vi "Set Configuration.vi"(8 "error in (no error)":errorcluster, 11 "Output Signal in":refnum<class "Output Signal.lvclass">) -> (0 "error out":errorcluster, 3 "Output Signal out":refnum<class "Output Signal.lvclass">)   [LabVIEW 2015, in "Output Signal.lvclass"]
uses:
  Output Signal.lvclass
  IO Class/Direction.ctl
  IO Class/IO Class.lvclass
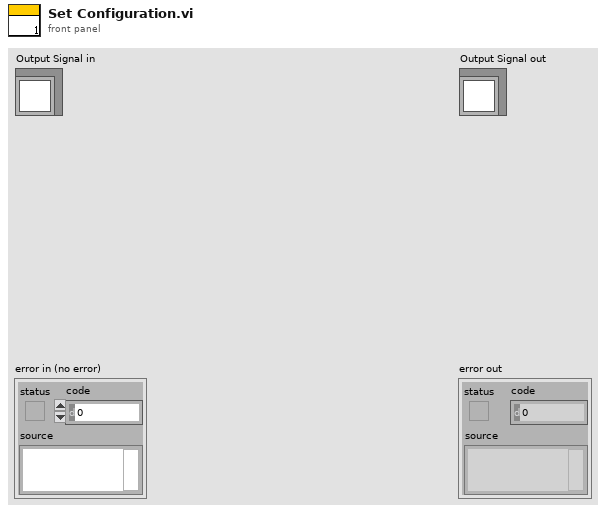
[diagram p1: front panel]
types:
  T1 = typedef "IO Class.lvclass/Direction.ctl" = cluster{"Direction":string}
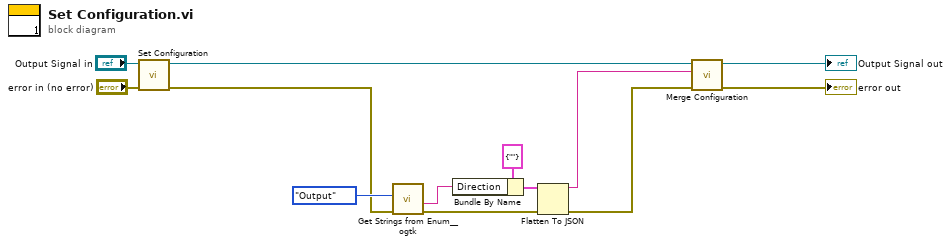
[diagram p0: block diagram]
diagram:
  n1 = call-parent "Set Configuration.vi"("error in (no error)"="error in (no error)", "IO Class in"="Output Signal in") -> ("error out"=w3:errorcluster, "IO Class out"=w2:refnum<class "Output Signal.lvclass">)  [unwired: 8 in]
  n2 = call <userlib>:"Get Strings from Enum__ogtk.vi"("error in (no error)"=w3, "Enum"=enum16{"Input", "Output"}."Output" ("Direction")) -> ("error out"=w8:errorcluster, "String Value"=w10:string)  [unwired: 6 in, 2 out]
  n3 = Bundle By Name(cluster=T1 {"Direction"=""} ("Cluster"), "Direction"=w10) -> (w9:T1)
  n4 = Flatten To JSON(anything=w9, error in (no error)=w8) -> (JSON string=w6:string, 11:w1:errorcluster)  [unwired: 1 in]
  n5 = call "Merge Configuration.vi"("error in (no error)"=w1, "Additional Configuration"=w6, "IO Class in"=w2) -> ("error out"=→"error out":errorcluster, "IO Class out"=→"Output Signal out":refnum<class "Output Signal.lvclass">)  [unwired: 7 in]
